vi "Stream Controller (FPGA).vi"() -> ()   [LabVIEW 2016]
doc: "Controls the generation and reception of data transferred from the Host to the FPGA.\nPort 0 receives data from the Port 0 TX Input DMA FIFO and transmits that data to Port 1.\nPort 1 receives data from the Port 1 TX Input DMA FIFO and transmits that data to Port 0."
uses:
  <instrlib>/_niInstr/Streaming/v1/Common/Stream State.ctl
  <vilib>/Platform/TimedLoop/XDataNode/timing_clust.ctl
  <vilib>/Platform/TimedLoop/XDataNode/nitl_modes.ctl
  <vilib>/Platform/TimedLoop/XDataNode/wakeup.ctl
  <instrlib>/_niInstr/CLIP Adapters/v1/FPGA/AXI4-Lite/FXP32 Address - FXP32 Data/Public/CLIP Resources.ctl
  <instrlib>/_niInstr/CLIP Adapters/v1/FPGA/AXI4-Lite/Address Space Collection/niInstr AXI4-Lite Address Space Collection v1 FPGA.lvclass
  C:/Program Files (x86)/National Instruments/LabVIEW 2016/instr.lib/_niInstr/Instruction Framework/v1/FPGA/Interfaces/Address Space Collection/Address Space Collection.lvclass
  <instrlib>/_niInstr/FIFO Register Bus/v1/FPGA/niInstr FIFO Register Bus v1 FPGA.lvclass
  C:/Program Files (x86)/National Instruments/LabVIEW 2016/instr.lib/_niInstr/Instruction Framework/v1/FPGA/Interfaces/Instruction Producer/Instruction Producer.lvclass
  <instrlib>/_niInstr/CLIP Adapters/v1/FPGA/AXI4-Stream/Reader FXP64x1/niInstr AXI4-Stream Reader FXP64x1 v1 FPGA.lvclass
  C:/Program Files (x86)/National Instruments/LabVIEW 2016/instr.lib/_niInstr/CLIP Adapters/v1/FPGA/AXI4-Stream/Reader/niInstr AXI4-Stream Reader v1 FPGA.lvclass
  <instrlib>/_niInstr/CLIP Adapters/v1/FPGA/AXI4-Stream/Writer FXP64x1/niInstr AXI4-Stream Writer FXP64x1 v1 FPGA.lvclass
  C:/Program Files (x86)/National Instruments/LabVIEW 2016/instr.lib/_niInstr/CLIP Adapters/v1/FPGA/AXI4-Stream/Writer/niInstr AXI4-Stream Writer v1 FPGA.lvclass
  <vilib>/rvi/Emulation/niFpgaSctlEmulationGetInTimedLoop.vi
  <vilib>/rvi/Emulation/niFpgaEmulationReportErrorSimple.vi
  <vilib>/rvi/Emulation/niFpgaGetClockAttributes.vi
  <vilib>/rvi/Emulation/niFpgaCriticalErrorInLSC.vi
  <instrlib>/_niInstr/Basic Elements/v1/FPGA/Private/Read U64 FIFO.vi
  <instrlib>/_niInstr/Basic Elements/v1/FPGA/Private/Write U64 FIFO.vi
  <vilib>/rvi/Emulation/niFpgaProcessEmulError.vi
  <vilib>/rvi/eio/common/nirviEmuTemplateMethod_errors.vi
  <vilib>/Platform/TimedLoop/XDataNode/XDataNode.xnode
  <vilib>/eio/EIONode/EIONode.xnode
  <vilib>/Platform/TimedLoop/XDataNode/XDNodeRunTimeDep.lvlib
  <instrlib>/_niInstr/CLIP Adapters/v1/FPGA/AXI4-Stream/Writer/niInstr AXI4-Stream Writer v1 FPGA.lvclass
  <instrlib>/_niInstr/CLIP Adapters/v1/FPGA/AXI4-Stream/Reader/niInstr AXI4-Stream Reader v1 FPGA.lvclass
  <instrlib>/_niInstr/Basic Elements/v1/FPGA/niInstr Basic Elements v1 FPGA.lvlib
  SubVIS/Aurora Stream (NI 6592R) (FPGA).lvlib
  <instrlib>/_niInstr/Streaming/v1/FPGA/niInstr Streaming v1 FPGA.lvlib
  <instrlib>/_niInstr/Streaming/v1/Common/niInstr Streaming v1 Common.lvlib
  <instrlib>/_niInstr/Instruction Framework/v1/FPGA/Top Level Bus/Register Configuration/Register Configuration.lvclass
  <instrlib>/_niInstr/CLIP Adapters/v1/FPGA/AXI4-Lite/FXP32 Address - FXP32 Data/niInstr AXI4-Lite - FXP32 Address - FXP32 Data v1 FPGA.lvclass
panel:
  out "Er.Port 3":u32
  out "Er.Port 2":u32
  out "Er.Port 1":u32
  out "Er.Port 0":u32
  in  "Simulated data":bool
  in  "Reset":bool
  out "Port 3 Link Reset":bool
  out "Port 1 Link Reset":bool
  in  "Port 3 PMA Init":bool
  in  "Port 1 PMA Init":bool
  out "fifo reg bus data 0":u64
  out "fifo reg bus status 0":u32
  in  "fifo reg bus ctrl 0":u32
  in  "Port 0 PMA Init":bool
  in  "Port 2 PMA Init":bool
  out "Port 0 Debug Info":T1
  out "Port 0 Link Reset":bool
  out "Port 2 Link Reset":bool
  out "sFrontEndConfig_Complete":bool
  out "Port 2 Debug Info":T1
  out "stream.state 5":T2
  out "stream.samples transferred 5":u64
  out "stream.metadata 5":u64
  in  "stream.num samples 5":u64
  in  "stream.request state 5":T2
  out "stream.state 4":T2
  out "stream.samples transferred 4":u64
  out "stream.metadata 4":u64
  in  "stream.num samples 4":u64
  in  "stream.request state 4":T2
  in  "stream.request state 0":T2
  in  "stream.num samples 0":u64
  out "stream.metadata 0":u64
  out "stream.samples transferred 0":u64
  out "stream.state 0":T2
  in  "stream.num samples 1":u64
  in  "stream.request state 1":T2
  out "stream.state 1":T2
  out "stream.samples transferred 1":u64
  out "stream.metadata 1":u64
  in  "stream.request state 6":T2
  in  "stream.num samples 6":u64
  out "stream.metadata 6":u64
  out "stream.samples transferred 6":u64
  out "stream.state 6":T2
  in  "stream.request state 7":T2
  in  "stream.num samples 7":u64
  out "stream.metadata 7":u64
  out "stream.samples transferred 7":u64
  out "stream.state 7":T2
  out "Port 3 Debug Info":T1
  in  "stream.request state 2":T2
  in  "stream.num samples 2":u64
  out "stream.metadata 2":u64
  out "stream.samples transferred 2":u64
  out "stream.state 2":T2
  in  "stream.request state 3":T2
  in  "stream.num samples 3":u64
  out "stream.metadata 3":u64
  out "stream.samples transferred 3":u64
  out "stream.state 3":T2
  out "Port 1 Debug Info":T1
  # "Port 0"
  # "Port 1"
  # "Port 2"
  # "Port 3"
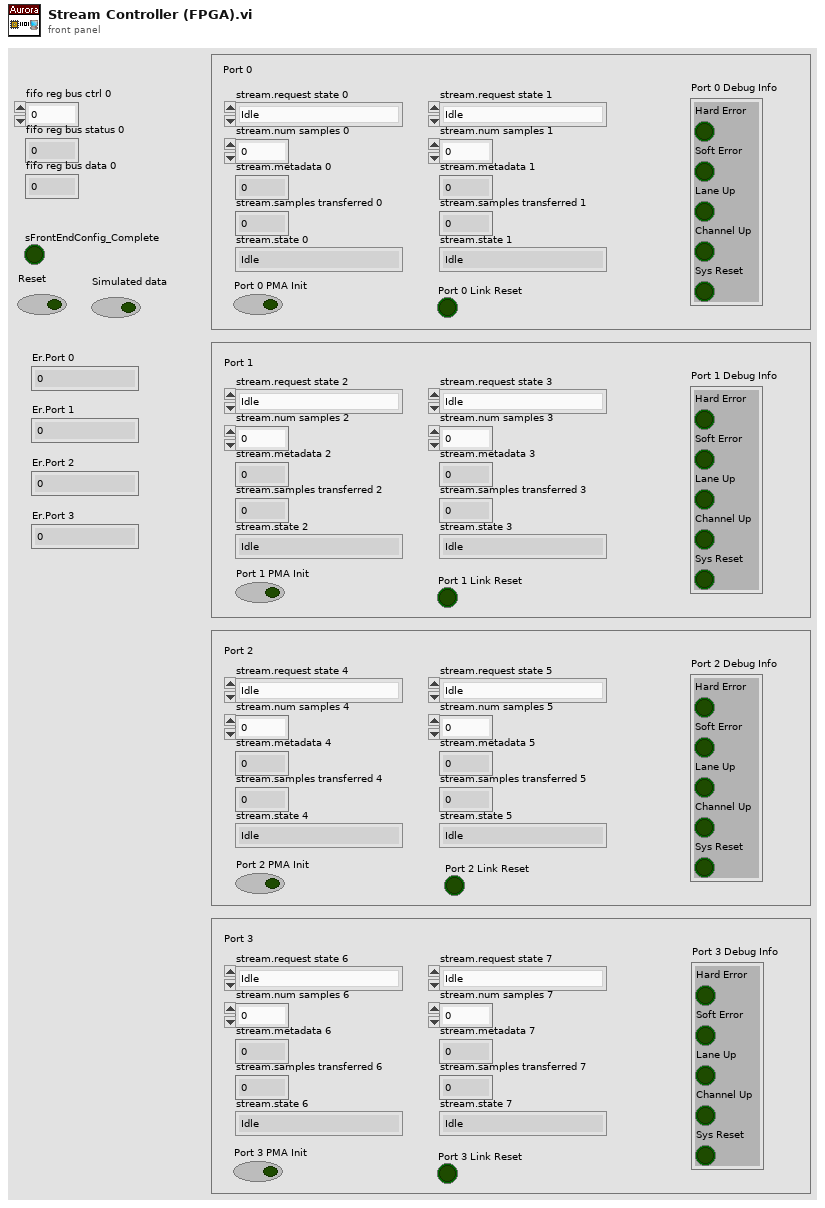
[diagram p1: front panel]
types:
  T1 = cluster{"Hard Error":bool, "Soft Error":bool, "Lane Up":bool, "Channel Up":bool, "Sys Reset":bool}
  T2 = typedef "niInstr Streaming v1 Common.lvlib/Stream State.ctl" = enum8{"Idle", "Finite Transfer", "Continuous", "Done", "Error", "Not Ready", "Cancel"}
  T3 = cluster{"Hard Error":refnum<k21>, "Soft Error":refnum<k21>, "Lane Up":refnum<k21>, "Channel Up":refnum<k21>, "Sys Reset":refnum<k21>}
  T4 = cluster{"m_axis_tvalid":refnum<k21>, "m_axis_tdata":refnum<k21>}
  T5 = cluster{"s_axis_tvalid":refnum<k21>, "s_axis_tdata":refnum<k21>, "s_axis_tready":refnum<k21>}
  T6 = typedef "niInstr AXI4-Lite - FXP32 Address - FXP32 Data v1 FPGA.lvclass/CLIP Resources.ctl" = cluster{"s_axi_araddr":refnum<k21>, "s_axi_arvalid":refnum<k21>, "s_axi_arready":refnum<k21>, "s_axi_rdata":refnum<k21>, "s_axi_rresp":refnum<k21>, "s_axi_rvalid":refnum<k21>, "s_axi_rready":refnum<k21>, "s_axi_awaddr":refnum<k21>, "s_axi_awvalid":refnum<k21>, "s_axi_awready":refnum<k21>, "s_axi_wdata":refnum<k21>, "s_axi_wstrb":refnum<k21>, "s_axi_wvalid":refnum<k21>, "s_axi_wready":refnum<k21>, "s_axi_bresp":refnum<k21>, "s_axi_bvalid":refnum<k21>, "s_axi_bready":refnum<k21>}
  T7 = typedef "XDNodeRunTimeDep.lvlib/timing_clust.ctl" = cluster{"Expected End [f-1]":u64, "Actual End [f-1]":u64, "Finished Late? [f-1]":bool, "Expected End [i-1]":u64, "Actual End [i-1]":u64, "Finished Late? [i-1]":bool, "Expected Start [i]":u64, "Actual Start [i]":u64, "Expected Start [f]":u64, "Actual Start [f]":u64, "Source Name":string, "Structure Name":string, "Period":i64, "Deadline":i64, "Offset":i64, "Start":i64, "Priority":i32, "Timeout":i32, "Mode":T8, "Wakeup Reason":T9, "Error":errorcluster, "Source Type":string, "Secondary Source Type":string, "Global End Time":u64, "Global Start Time":u64, "Frame Duration":u64, "Iteration Duration":u64, "Assigned CPU":i32, "I/O Scan Engine Mode":u32}
  T8 = typedef "XDNodeRunTimeDep.lvlib/nitl_modes.ctl" = enum32{"No Change", "Process missed periods, maintain original phase", "Discard missed periods, maintain original phase", "Process missed periods, ignore original phase", "Discard missed periods, ignore original phase"}
  T9 = typedef "XDNodeRunTimeDep.lvlib/wakeup.ctl" = enum32{"Normal", "Aborted", "Asynchronous wakeup", "Timing source error", "Timed loop error", "Timeout"}
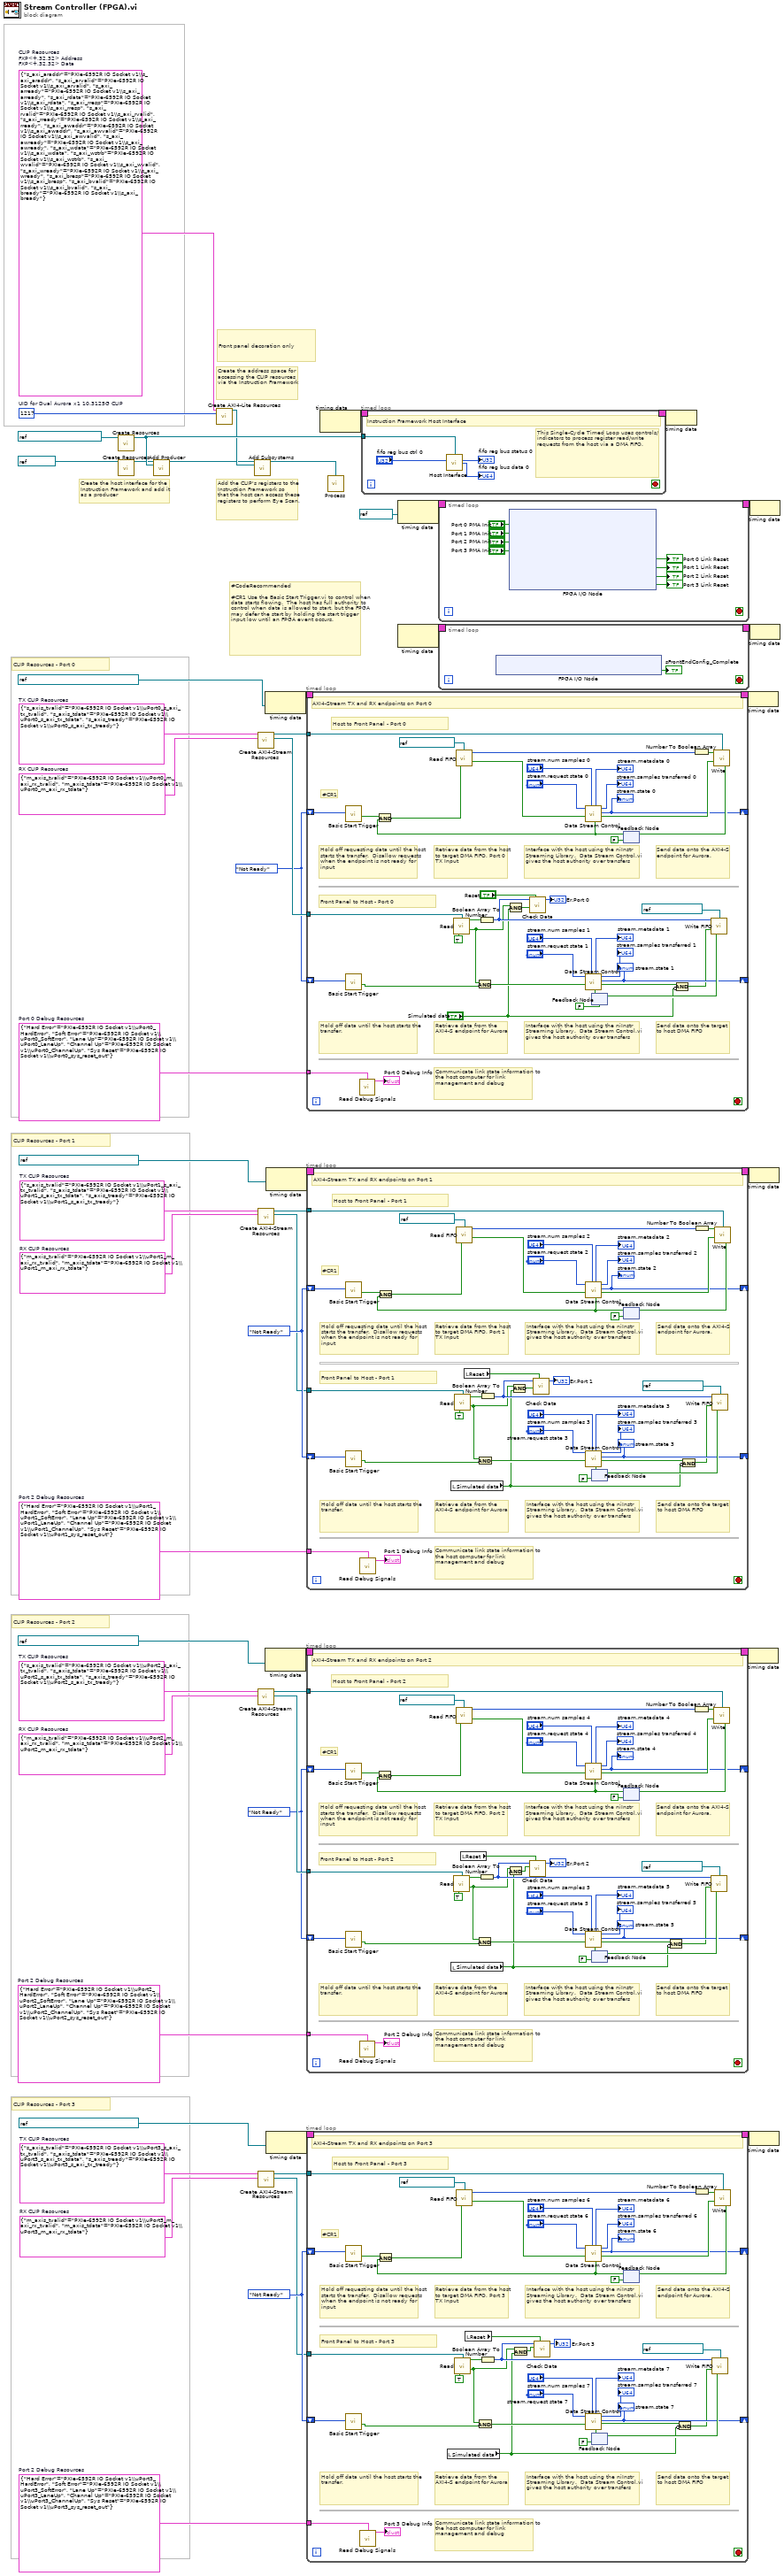
[diagram p0: block diagram]
diagram:
  w10 = T3 {"Hard Error"="PXIe-6592R IO Socket v1\\uPort3_HardError", "Soft Error"="PXIe-6592R IO Socket v1\\uPort3_SoftError", "Lane Up"="PXIe-6592R IO Socket v1\\uPort3_LaneUp", "Channel Up"="PXIe-6592R IO Socket v1\\uPort3_ChannelUp", "Sys Reset"="PXIe-6592R IO Socket v1\\uPort3_sys_reset_out"}  # Port 2 Debug Resources
  w9 = Stream_State."Not Ready" ("stream.state 0")
  w5 = T4 {"m_axis_tvalid"="PXIe-6592R IO Socket v1\\uPort3_m_axi_rx_tvalid", "m_axis_tdata"="PXIe-6592R IO Socket v1\\uPort3_m_axi_rx_tdata"}  # RX CLIP Resources
  w4 = T5 {"s_axis_tvalid"="PXIe-6592R IO Socket v1\\uPort3_s_axi_tx_tvalid", "s_axis_tdata"="PXIe-6592R IO Socket v1\\uPort3_s_axi_tx_tdata", "s_axis_tready"="PXIe-6592R IO Socket v1\\uPort3_s_axi_tx_tready"}  # TX CLIP Resources
  w19 = T3 {"Hard Error"="PXIe-6592R IO Socket v1\\uPort1_HardError", "Soft Error"="PXIe-6592R IO Socket v1\\uPort1_SoftError", "Lane Up"="PXIe-6592R IO Socket v1\\uPort1_LaneUp", "Channel Up"="PXIe-6592R IO Socket v1\\uPort1_ChannelUp", "Sys Reset"="PXIe-6592R IO Socket v1\\uPort1_sys_reset_out"}  # Port 2 Debug Resources
  w18 = Stream_State."Not Ready" ("stream.state 0")
  w14 = T4 {"m_axis_tvalid"="PXIe-6592R IO Socket v1\\uPort1_m_axi_rx_tvalid", "m_axis_tdata"="PXIe-6592R IO Socket v1\\uPort1_m_axi_rx_tdata"}  # RX CLIP Resources
  w13 = T5 {"s_axis_tvalid"="PXIe-6592R IO Socket v1\\uPort1_s_axi_tx_tvalid", "s_axis_tdata"="PXIe-6592R IO Socket v1\\uPort1_s_axi_tx_tdata", "s_axis_tready"="PXIe-6592R IO Socket v1\\uPort1_s_axi_tx_tready"}  # TX CLIP Resources
  w33 = u16 1217  # UID for Dual Aurora x1 10.3125G CLIP
  w34 = T6 {"s_axi_araddr"="PXIe-6592R IO Socket v1\\s_axi_araddr", "s_axi_arvalid"="PXIe-6592R IO Socket v1\\s_axi_arvalid", "s_axi_arready"="PXIe-6592R IO Socket v1\\s_axi_arready", "s_axi_rdata"="PXIe-6592R IO Socket v1\\s_axi_rdata", "s_axi_rresp"="PXIe-6592R IO Socket v1\\s_axi_rresp", "s_axi_rvalid"="PXIe-6592R IO Socket v1\\s_axi_rvalid", "s_axi_rready"="PXIe-6592R IO Socket v1\\s_axi_rready", "s_axi_awaddr"="PXIe-6592R IO Socket v1\\s_axi_awaddr", "s_axi_awvalid"="PXIe-6592R IO Socket v1\\s_axi_awvalid", "s_axi_awready"="PXIe-6592R IO Socket v1\\s_axi_awready", "s_axi_wdata"="PXIe-6592R IO Socket v1\\s_axi_wdata", "s_axi_wstrb"="PXIe-6592R IO Socket v1\\s_axi_wstrb", "s_axi_wvalid"="PXIe-6592R IO Socket v1\\s_axi_wvalid", "s_axi_wready"="PXIe-6592R IO Socket v1\\s_axi_wready", "s_axi_bresp"="PXIe-6592R IO Socket v1\\s_axi_bresp", "s_axi_bvalid"="PXIe-6592R IO Socket v1\\s_axi_bvalid", "s_axi_bready"="PXIe-6592R IO Socket v1\\s_axi_bready"}  # CLIP Resources FXP<+,32,32> Address FXP<+,32,32> Data
  w22 = T3 {"Hard Error"="PXIe-6592R IO Socket v1\\uPort2_HardError", "Soft Error"="PXIe-6592R IO Socket v1\\uPort2_SoftError", "Lane Up"="PXIe-6592R IO Socket v1\\uPort2_LaneUp", "Channel Up"="PXIe-6592R IO Socket v1\\uPort2_ChannelUp", "Sys Reset"="PXIe-6592R IO Socket v1\\uPort2_sys_reset_out"}  # Port 2 Debug Resources
  w40 = T3 {"Hard Error"="PXIe-6592R IO Socket v1\\uPort0_HardError", "Soft Error"="PXIe-6592R IO Socket v1\\uPort0_SoftError", "Lane Up"="PXIe-6592R IO Socket v1\\uPort0_LaneUp", "Channel Up"="PXIe-6592R IO Socket v1\\uPort0_ChannelUp", "Sys Reset"="PXIe-6592R IO Socket v1\\uPort0_sys_reset_out"}  # Port 0 Debug Resources
  w23 = Stream_State."Not Ready" ("stream.state 0")
  w41 = Stream_State."Not Ready" ("stream.state 0")
  w45 = T4 {"m_axis_tvalid"="PXIe-6592R IO Socket v1\\uPort2_m_axi_rx_tvalid", "m_axis_tdata"="PXIe-6592R IO Socket v1\\uPort2_m_axi_rx_tdata"}  # RX CLIP Resources
  w46 = T5 {"s_axis_tvalid"="PXIe-6592R IO Socket v1\\uPort2_s_axi_tx_tvalid", "s_axis_tdata"="PXIe-6592R IO Socket v1\\uPort2_s_axi_tx_tdata", "s_axis_tready"="PXIe-6592R IO Socket v1\\uPort2_s_axi_tx_tready"}  # TX CLIP Resources
  w47 = T4 {"m_axis_tvalid"="PXIe-6592R IO Socket v1\\uPort0_m_axi_rx_tvalid", "m_axis_tdata"="PXIe-6592R IO Socket v1\\uPort0_m_axi_rx_tdata"}  # RX CLIP Resources
  w48 = T5 {"s_axis_tvalid"="PXIe-6592R IO Socket v1\\uPort0_s_axi_tx_tvalid", "s_axis_tdata"="PXIe-6592R IO Socket v1\\uPort0_s_axi_tx_tdata", "s_axis_tready"="PXIe-6592R IO Socket v1\\uPort0_s_axi_tx_tready"}  # TX CLIP Resources
  # "CLIP Resources - Port 3"
  # "CLIP Resources - Port 1"
  # "CLIP Resources - Port 2"
  # "CLIP Resources - Port 0"
  # "#CodeRecommended\n\n#CR1 Use the Basic Start Trigger.vi to control when data starts flowing.  The host has full authority to control when data is allowed to start, but the FPGA may defer the start by holding the start trigger input low until an FPGA event occurs."
  # "Add the CLIP's registers to the Instruction Framework so\nthat the host can access these registers to perform Eye Scan."
  # "Create the host interface for the Instruction Framework and add it as a producer"
  # "Create the address space for accessing the CLIP resources via the Instruction Framework"
  # "Front panel decoration only"
  n1 = call <instrlib>:"Create Resources.vi"("instruction fifo"=refnum<k21> "reg.host instruction fifo 0" ("FIFO")) -> ("fifo register bus"=w35:refnum<class "niInstr FIFO Register Bus v1 FPGA.lvclass">)  [unwired: 14 in]
  n2 = call <instrlib>:"Create Resources.vi"("register clock"=refnum<k21> "100MHz" ("Source Name")) -> ("register configuration"=w31:refnum<class "Register Configuration.lvclass">)  [unwired: 14 in]
  n3 = call <instrlib>:"Add Producer.vi"("register configuration in"=w31, "instruction producer"=w35) -> ("register configuration out"=w30:refnum<class "Register Configuration.lvclass">)  [unwired: 13 in]
  n4 = call "Create AXI4-Lite Resources.vi"("CLIP Resources\nFXP<+,32,32> Address\nFXP<+,32,32> Data"=w34, "UID for Dual Aurora x1 10.3125G CLIP"=w33) -> ("niInstr AXI4-Lite Address Space Collection v1 FPGA out"=w32:refnum<class "niInstr AXI4-Lite Address Space Collection v1 FPGA.lvclass">)  [unwired: 13 in]
  n5 = call <instrlib>:"Add Subsystems.vi"("register configuration in"=w30, "subsystems"=w32) -> ("register configuration out"=w29:refnum<class "Register Configuration.lvclass">)  [unwired: 13 in]
  n6 = call "Create AXI4-Stream Resources.vi"("RX CLIP Resources"=w47, "TX CLIP Resources"=w48) -> ("RX niInstr AXI4-Stream Reader FXP64x1 v1 FPGA out"=w42:refnum<class "niInstr AXI4-Stream Reader FXP64x1 v1 FPGA.lvclass">, "TX niInstr AXI4-Stream Reader FXP64x1 v1 FPGA out"=w49:refnum<class "niInstr AXI4-Stream Writer FXP64x1 v1 FPGA.lvclass">)  [unwired: 8 in]
  n7 = call "Create AXI4-Stream Resources.vi"("RX CLIP Resources"=w45, "TX CLIP Resources"=w46) -> ("RX niInstr AXI4-Stream Reader FXP64x1 v1 FPGA out"=w24:refnum<class "niInstr AXI4-Stream Reader FXP64x1 v1 FPGA.lvclass">, "TX niInstr AXI4-Stream Reader FXP64x1 v1 FPGA out"=w25:refnum<class "niInstr AXI4-Stream Writer FXP64x1 v1 FPGA.lvclass">)  [unwired: 8 in]
  n8 = call "Create AXI4-Stream Resources.vi"("RX CLIP Resources"=w14, "TX CLIP Resources"=w13) -> ("RX niInstr AXI4-Stream Reader FXP64x1 v1 FPGA out"=w17:refnum<class "niInstr AXI4-Stream Reader FXP64x1 v1 FPGA.lvclass">, "TX niInstr AXI4-Stream Reader FXP64x1 v1 FPGA out"=w16:refnum<class "niInstr AXI4-Stream Writer FXP64x1 v1 FPGA.lvclass">)  [unwired: 8 in]
  n9 = call "Create AXI4-Stream Resources.vi"("RX CLIP Resources"=w5, "TX CLIP Resources"=w4) -> ("RX niInstr AXI4-Stream Reader FXP64x1 v1 FPGA out"=w8:refnum<class "niInstr AXI4-Stream Reader FXP64x1 v1 FPGA.lvclass">, "TX niInstr AXI4-Stream Reader FXP64x1 v1 FPGA out"=w7:refnum<class "niInstr AXI4-Stream Writer FXP64x1 v1 FPGA.lvclass">)  [unwired: 8 in]
  n10 = node-c288(refnum<k21> "PXIe-6592R IO Socket v1\\Port0_UserClk" ("Source Name")) -> (w52:T7)
  n11 = node-c288(refnum<k21> "PXIe-6592R IO Socket v1\\Port2_UserClk" ("Source Name")) -> (w28:T7)
  n12 = node-c288(refnum<k21> "PXIe-6592R IO Socket v1\\Port1_UserClk" ("Source Name")) -> (w21:T7)
  n13 = node-c288(refnum<k21> "PXIe-6592R IO Socket v1\\Port3_UserClk" ("Source Name")) -> (w12:T7)
  n14 = timed-loop {
    timing: w52 -> [_]
    timing-out: [_] -> w51
    tunnel: w49 -> [w93]
    tunnel: w42 -> [w92]
    shift-right: [w84] -> _
    shift-left: w41 -> [w79]
    shift-right: [w66] -> _
    shift-left: w41 -> [w72]
    tunnel: w40 -> [w64]
    stop <- _ stop-if-true
    # "#CR1"
    # "Communicate link state information to the host computer for link management and debug"
    # "Send data onto the target to host DMA FIFO"
    # "Interface with the host using the niInstr Streaming Library.  Data Stream Control.vi gives the host authority over transfers"
    # "Retrieve data from the AXI4-S endpoint for Aurora"
    # "Hold off data until the host starts the transfer."
    # "Send data onto the AXI4-S endpoint for Aurora."
    # "Interface with the host using the niInstr Streaming Library.  Data Stream Control.vi gives the host authority over transfers"
    # "Retrieve data from the host to target DMA FIFO, Port 0 TX Input"
    # "Hold off requesting data until the host starts the transfer.  Disallow requests when the endpoint is not ready for input"
    # "Front Panel to Host - Port 0"
    # "Host to Front Panel - Port 0"
    # "AXI4-Stream TX and RX endpoints on Port 0"
    n15 = call <instrlib>:"Basic Start Trigger.vi"("stream.state"=w79) -> ("data valid"=w78:bool)  [unwired: 10 in]
    n16 = call <instrlib>:"Basic Start Trigger.vi"("stream.state"=w72) -> ("data valid"=w71:bool)  [unwired: 10 in]
    n17 = call "Read Debug Signals.vi"("Debug CLIP Resources"=w64) -> ("Debug Info"=→"Port 0 Debug Info":T1)  [unwired: 14 in]
    n18 = call <instrlib>:"Read.vi"("niInstr AXI4-Stream Reader v1 FPGA in"=w92, "ready for output"=TRUE) -> ("tdata"=w88:bool[], "output valid"=w56:bool)  [unwired: 8 in, 4 out]
    n19 = And(x=w56, y=w71) -> (x .and. y?=w65:bool)
    n20 = Boolean Array To Number(Boolean array=w88) -> (number=w59:u64)
    n21 = Compound Arithmetic op=AND(w56, "Simulated data") -> (w55:bool)
    n22 = call "Check Data.vi"("reset"="Reset", "Input valid"=w55, "IQ Stream"=w59) -> ("errors"=→"Er.Port 0":u32)  [unwired: 8 in]
    n23 = feedback #1(FALSE ("ready for input")) -> (w73:bool)
    n24 = call <instrlib>:"Data Stream Control.vi"("ready for input?"=w73, "stream.num samples 0"="stream.num samples 1", "data valid"=w65, "stream.request state 0"="stream.request state 1") -> ("send data"=w58:bool, "stream.state 0"=w66:T2, "stream.samples transferred 0"=→"stream.samples transferred 1":u64, "stream.metadata 0"=→"stream.metadata 1":u64)  [unwired: 3 in, 1 out]
    "stream.state 1" <- w66
    n25 = feedback #2(FALSE ("ready for input")) -> (w77:bool)
    n26 = And(x=w78, y=w77) -> (x .and. y?=w76:bool)
    n27 = call-poly <instrlib>:"Read FIFO.vi"("fifo"=refnum<k21> "Port 0 TX Input", "ready for output"=w76) -> ("output data"=w86:u64, "output valid"=w75:bool)  [unwired: 12 in]
    n28 = call <instrlib>:"Data Stream Control.vi"("ready for input?"=w77, "stream.num samples 0"="stream.num samples 0", "data valid"=w75, "stream.request state 0"="stream.request state 0") -> ("send data"=w85:bool, "stream.state 0"=w84:T2, "stream.samples transferred 0"=→"stream.samples transferred 0":u64, "stream.metadata 0"=→"stream.metadata 0":u64)  [unwired: 3 in, 1 out]
    "stream.state 0" <- w84
    n29 = Compound Arithmetic op=AND(w58, invert "Simulated data") -> (w57:bool)
    n30 = Number To Boolean Array(number=w86) -> (Boolean array=w90:bool[])
    n31 = call-poly <instrlib>:"Write FIFO.vi"("input data"=w59, "fifo"=refnum<k21> "Port 0 RX Output", "input valid"=w57) -> ("ready for input"=w74:bool)  [unwired: 12 in]
    n32 = feedback-in #1(w74) -> ()
    n33 = call <instrlib>:"Write.vi"("tdata"=w90, "niInstr AXI4-Stream Writer v1 FPGA in"=w93, "input valid"=w85) -> ("ready for input"=w87:bool)  [unwired: 12 in]
    n34 = feedback-in #2(w87) -> ()
  }
  n35 = timed-loop {
    timing: w28 -> [_]
    timing-out: [_] -> w27
    tunnel: w25 -> [w137]
    tunnel: w24 -> [w136]
    shift-right: [w128] -> _
    shift-left: w23 -> [w123]
    shift-right: [w110] -> _
    shift-left: w23 -> [w116]
    tunnel: w22 -> [w108]
    stop <- _ stop-if-true
    # "#CR1"
    # "Communicate link state information to the host computer for link management and debug"
    # "Send data onto the target to host DMA FIFO"
    # "Interface with the host using the niInstr Streaming Library.  Data Stream Control.vi gives the host authority over transfers"
    # "Retrieve data from the AXI4-S endpoint for Aurora"
    # "Hold off data until the host starts the transfer."
    # "Send data onto the AXI4-S endpoint for Aurora."
    # "Interface with the host using the niInstr Streaming Library.  Data Stream Control.vi gives the host authority over transfers"
    # "Retrieve data from the host to target DMA FIFO, Port 2 TX Input"
    # "Hold off requesting data until the host starts the transfer.  Disallow requests when the endpoint is not ready for input"
    # "Front Panel to Host - Port 2"
    # "Host to Front Panel - Port 2"
    # "AXI4-Stream TX and RX endpoints on Port 2"
    n36 = call <instrlib>:"Basic Start Trigger.vi"("stream.state"=w123) -> ("data valid"=w122:bool)  [unwired: 10 in]
    n37 = call <instrlib>:"Basic Start Trigger.vi"("stream.state"=w116) -> ("data valid"=w115:bool)  [unwired: 10 in]
    n38 = call "Read Debug Signals.vi"("Debug CLIP Resources"=w108) -> ("Debug Info"=→"Port 2 Debug Info":T1)  [unwired: 14 in]
    n39 = local read "Simulated data"() -> (w98:bool)
    n40 = call <instrlib>:"Read.vi"("niInstr AXI4-Stream Reader v1 FPGA in"=w136, "ready for output"=TRUE) -> ("tdata"=w132:bool[], "output valid"=w101:bool)  [unwired: 8 in, 4 out]
    n41 = local read "Reset"() -> (w103:bool)
    n42 = And(x=w101, y=w115) -> (x .and. y?=w109:bool)
    n43 = Boolean Array To Number(Boolean array=w132) -> (number=w102:u64)
    n44 = Compound Arithmetic op=AND(w101, w98) -> (w100:bool)
    n45 = call "Check Data.vi"("reset"=w103, "Input valid"=w100, "IQ Stream"=w102) -> ("errors"=→"Er.Port 2":u32)  [unwired: 8 in]
    n46 = feedback #3(FALSE ("ready for input")) -> (w117:bool)
    n47 = call <instrlib>:"Data Stream Control.vi"("ready for input?"=w117, "stream.num samples 0"="stream.num samples 5", "data valid"=w109, "stream.request state 0"="stream.request state 5") -> ("send data"=w99:bool, "stream.state 0"=w110:T2, "stream.samples transferred 0"=→"stream.samples transferred 5":u64, "stream.metadata 0"=→"stream.metadata 5":u64)  [unwired: 3 in, 1 out]
    "stream.state 5" <- w110
    n48 = feedback #4(FALSE ("ready for input")) -> (w121:bool)
    n49 = And(x=w122, y=w121) -> (x .and. y?=w120:bool)
    n50 = call-poly <instrlib>:"Read FIFO.vi"("fifo"=refnum<k21> "Port 2 TX Input", "ready for output"=w120) -> ("output data"=w130:u64, "output valid"=w119:bool)  [unwired: 12 in]
    n51 = call <instrlib>:"Data Stream Control.vi"("ready for input?"=w121, "stream.num samples 0"="stream.num samples 4", "data valid"=w119, "stream.request state 0"="stream.request state 4") -> ("send data"=w129:bool, "stream.state 0"=w128:T2, "stream.samples transferred 0"=→"stream.samples transferred 4":u64, "stream.metadata 0"=→"stream.metadata 4":u64)  [unwired: 3 in, 1 out]
    "stream.state 4" <- w128
    n52 = Compound Arithmetic op=AND(w99, invert w98) -> (w97:bool)
    n53 = Number To Boolean Array(number=w130) -> (Boolean array=w134:bool[])
    n54 = call-poly <instrlib>:"Write FIFO.vi"("input data"=w102, "fifo"=refnum<k21> "Port 2 RX Output", "input valid"=w97) -> ("ready for input"=w118:bool)  [unwired: 12 in]
    n55 = feedback-in #3(w118) -> ()
    n56 = call <instrlib>:"Write.vi"("tdata"=w134, "niInstr AXI4-Stream Writer v1 FPGA in"=w137, "input valid"=w129) -> ("ready for input"=w131:bool)  [unwired: 12 in]
    n57 = feedback-in #4(w131) -> ()
  }
  n58 = timed-loop {
    timing: w21 -> [_]
    timing-out: [_] -> w20
    tunnel: w16 -> [w181]
    tunnel: w17 -> [w180]
    shift-right: [w172] -> _
    shift-left: w18 -> [w167]
    shift-right: [w154] -> _
    shift-left: w18 -> [w160]
    tunnel: w19 -> [w152]
    stop <- _ stop-if-true
    # "#CR1"
    # "Communicate link state information to the host computer for link management and debug"
    # "Send data onto the target to host DMA FIFO"
    # "Interface with the host using the niInstr Streaming Library.  Data Stream Control.vi gives the host authority over transfers"
    # "Retrieve data from the AXI4-S endpoint for Aurora"
    # "Hold off data until the host starts the transfer."
    # "Send data onto the AXI4-S endpoint for Aurora."
    # "Interface with the host using the niInstr Streaming Library.  Data Stream Control.vi gives the host authority over transfers"
    # "Retrieve data from the host to target DMA FIFO, Port 1 TX Input"
    # "Hold off requesting data until the host starts the transfer.  Disallow requests when the endpoint is not ready for input"
    # "Front Panel to Host - Port 1"
    # "Host to Front Panel - Port 1"
    # "AXI4-Stream TX and RX endpoints on Port 1"
    n59 = call <instrlib>:"Basic Start Trigger.vi"("stream.state"=w167) -> ("data valid"=w166:bool)  [unwired: 10 in]
    n60 = call <instrlib>:"Basic Start Trigger.vi"("stream.state"=w160) -> ("data valid"=w159:bool)  [unwired: 10 in]
    n61 = call "Read Debug Signals.vi"("Debug CLIP Resources"=w152) -> ("Debug Info"=→"Port 1 Debug Info":T1)  [unwired: 14 in]
    n62 = local read "Simulated data"() -> (w141:bool)
    n63 = call <instrlib>:"Read.vi"("niInstr AXI4-Stream Reader v1 FPGA in"=w180, "ready for output"=TRUE) -> ("tdata"=w176:bool[], "output valid"=w144:bool)  [unwired: 8 in, 4 out]
    n64 = local read "Reset"() -> (w146:bool)
    n65 = And(x=w144, y=w159) -> (x .and. y?=w153:bool)
    n66 = Boolean Array To Number(Boolean array=w176) -> (number=w145:u64)
    n67 = Compound Arithmetic op=AND(w144, w141) -> (w148:bool)
    n68 = call "Check Data.vi"("reset"=w146, "Input valid"=w148, "IQ Stream"=w145) -> ("errors"=→"Er.Port 1":u32)  [unwired: 8 in]
    n69 = feedback #5(FALSE ("ready for input")) -> (w161:bool)
    n70 = call <instrlib>:"Data Stream Control.vi"("ready for input?"=w161, "stream.num samples 0"="stream.num samples 3", "data valid"=w153, "stream.request state 0"="stream.request state 3") -> ("send data"=w143:bool, "stream.state 0"=w154:T2, "stream.samples transferred 0"=→"stream.samples transferred 3":u64, "stream.metadata 0"=→"stream.metadata 3":u64)  [unwired: 3 in, 1 out]
    "stream.state 3" <- w154
    n71 = feedback #6(FALSE ("ready for input")) -> (w165:bool)
    n72 = And(x=w166, y=w165) -> (x .and. y?=w164:bool)
    n73 = call-poly <instrlib>:"Read FIFO.vi"("fifo"=refnum<k21> "Port 1 TX Input", "ready for output"=w164) -> ("output data"=w174:u64, "output valid"=w163:bool)  [unwired: 12 in]
    n74 = call <instrlib>:"Data Stream Control.vi"("ready for input?"=w165, "stream.num samples 0"="stream.num samples 2", "data valid"=w163, "stream.request state 0"="stream.request state 2") -> ("send data"=w173:bool, "stream.state 0"=w172:T2, "stream.samples transferred 0"=→"stream.samples transferred 2":u64, "stream.metadata 0"=→"stream.metadata 2":u64)  [unwired: 3 in, 1 out]
    "stream.state 2" <- w172
    n75 = Compound Arithmetic op=AND(w143, invert w141) -> (w142:bool)
    n76 = Number To Boolean Array(number=w174) -> (Boolean array=w178:bool[])
    n77 = call-poly <instrlib>:"Write FIFO.vi"("input data"=w145, "fifo"=refnum<k21> "Port 1 RX Output", "input valid"=w142) -> ("ready for input"=w162:bool)  [unwired: 12 in]
    n78 = feedback-in #5(w162) -> ()
    n79 = call <instrlib>:"Write.vi"("tdata"=w178, "niInstr AXI4-Stream Writer v1 FPGA in"=w181, "input valid"=w173) -> ("ready for input"=w175:bool)  [unwired: 12 in]
    n80 = feedback-in #6(w175) -> ()
  }
  n81 = timed-loop {
    timing: w12 -> [_]
    timing-out: [_] -> w11
    tunnel: w7 -> [w225]
    tunnel: w8 -> [w224]
    shift-right: [w216] -> _
    shift-left: w9 -> [w211]
    shift-right: [w198] -> _
    shift-left: w9 -> [w204]
    tunnel: w10 -> [w196]
    stop <- _ stop-if-true
    # "#CR1"
    # "Communicate link state information to the host computer for link management and debug"
    # "Send data onto the target to host DMA FIFO"
    # "Interface with the host using the niInstr Streaming Library.  Data Stream Control.vi gives the host authority over transfers"
    # "Retrieve data from the AXI4-S endpoint for Aurora"
    # "Hold off data until the host starts the transfer."
    # "Send data onto the AXI4-S endpoint for Aurora."
    # "Interface with the host using the niInstr Streaming Library.  Data Stream Control.vi gives the host authority over transfers"
    # "Retrieve data from the host to target DMA FIFO, Port 3 TX Input"
    # "Hold off requesting data until the host starts the transfer.  Disallow requests when the endpoint is not ready for input"
    # "Front Panel to Host - Port 3"
    # "Host to Front Panel - Port 3"
    # "AXI4-Stream TX and RX endpoints on Port 3"
    n82 = call <instrlib>:"Basic Start Trigger.vi"("stream.state"=w211) -> ("data valid"=w210:bool)  [unwired: 10 in]
    n83 = call <instrlib>:"Basic Start Trigger.vi"("stream.state"=w204) -> ("data valid"=w203:bool)  [unwired: 10 in]
    n84 = call "Read Debug Signals.vi"("Debug CLIP Resources"=w196) -> ("Debug Info"=→"Port 3 Debug Info":T1)  [unwired: 14 in]
    n85 = local read "Simulated data"() -> (w186:bool)
    n86 = call <instrlib>:"Read.vi"("niInstr AXI4-Stream Reader v1 FPGA in"=w224, "ready for output"=TRUE) -> ("tdata"=w220:bool[], "output valid"=w189:bool)  [unwired: 8 in, 4 out]
    n87 = local read "Reset"() -> (w191:bool)
    n88 = And(x=w189, y=w203) -> (x .and. y?=w197:bool)
    n89 = Boolean Array To Number(Boolean array=w220) -> (number=w190:u64)
    n90 = Compound Arithmetic op=AND(w189, w186) -> (w188:bool)
    n91 = call "Check Data.vi"("reset"=w191, "Input valid"=w188, "IQ Stream"=w190) -> ("errors"=→"Er.Port 3":u32)  [unwired: 8 in]
    n92 = feedback #7(FALSE ("ready for input")) -> (w205:bool)
    n93 = call <instrlib>:"Data Stream Control.vi"("ready for input?"=w205, "stream.num samples 0"="stream.num samples 7", "data valid"=w197, "stream.request state 0"="stream.request state 7") -> ("send data"=w187:bool, "stream.state 0"=w198:T2, "stream.samples transferred 0"=→"stream.samples transferred 7":u64, "stream.metadata 0"=→"stream.metadata 7":u64)  [unwired: 3 in, 1 out]
    "stream.state 7" <- w198
    n94 = feedback #8(FALSE ("ready for input")) -> (w209:bool)
    n95 = And(x=w210, y=w209) -> (x .and. y?=w208:bool)
    n96 = call-poly <instrlib>:"Read FIFO.vi"("fifo"=refnum<k21> "Port 3 TX Input", "ready for output"=w208) -> ("output data"=w218:u64, "output valid"=w207:bool)  [unwired: 12 in]
    n97 = call <instrlib>:"Data Stream Control.vi"("ready for input?"=w209, "stream.num samples 0"="stream.num samples 6", "data valid"=w207, "stream.request state 0"="stream.request state 6") -> ("send data"=w217:bool, "stream.state 0"=w216:T2, "stream.samples transferred 0"=→"stream.samples transferred 6":u64, "stream.metadata 0"=→"stream.metadata 6":u64)  [unwired: 3 in, 1 out]
    "stream.state 6" <- w216
    n98 = Compound Arithmetic op=AND(w187, invert w186) -> (w185:bool)
    n99 = Number To Boolean Array(number=w218) -> (Boolean array=w222:bool[])
    n100 = call-poly <instrlib>:"Write FIFO.vi"("input data"=w190, "fifo"=refnum<k21> "Port 3 RX Output", "input valid"=w185) -> ("ready for input"=w206:bool)  [unwired: 12 in]
    n101 = feedback-in #7(w206) -> ()
    n102 = call <instrlib>:"Write.vi"("tdata"=w222, "niInstr AXI4-Stream Writer v1 FPGA in"=w225, "input valid"=w217) -> ("ready for input"=w219:bool)  [unwired: 12 in]
    n103 = feedback-in #8(w219) -> ()
  }
  n104 = node-c288() -> (w39:T7)  [unwired: 1 in]
  n105 = call <instrlib>:"Process.vi"("register configuration"=w29) -> ()  [unwired: 15 in]
  n106 = timed-loop {
    timing: w39 -> [_]
    timing-out: [_] -> w38
    tunnel: w35 -> [w229]
    stop <- _ stop-if-true
    # "This Single-Cycle Timed Loop uses controls/indicators to process register read/write requests from the host via a DMA FIFO."
    # "Instruction Framework Host Interface"
    n107 = call <instrlib>:"Host Interface.vi"("fifo register bus"=w229, "fifo reg bus ctrl 0"="fifo reg bus ctrl 0") -> ("fifo reg bus status 0"=→"fifo reg bus status 0":u32, "fifo reg bus data 0"=→"fifo reg bus data 0":u64)  [unwired: 12 in]
  }
  n108 = node-c288(refnum<k21> "50MHz" ("Source Name")) -> (w44:T7)
  n109 = node-c288() -> (w3:T7)  [unwired: 1 in]
  n110 = timed-loop {
    timing: w44 -> [_]
    timing-out: [_] -> w43
    stop <- _ stop-if-true
    n111 = xnode "FPGA I/O Node"("PXIe-6592R IO Socket v1\\cPort0_PMA_Init"="Port 0 PMA Init", "PXIe-6592R IO Socket v1\\cPort1_PMA_Init"="Port 1 PMA Init", "PXIe-6592R IO Socket v1\\cPort2_PMA_Init"="Port 2 PMA Init", "PXIe-6592R IO Socket v1\\cPort3_PMA_Init"="Port 3 PMA Init") -> ("PXIe-6592R IO Socket v1\\cPort0_link_reset_out"=→"Port 0 Link Reset":bool, "PXIe-6592R IO Socket v1\\cPort1_link_reset_out"=→"Port 1 Link Reset":bool, "PXIe-6592R IO Socket v1\\cPort2_link_reset_out"=→"Port 2 Link Reset":bool, "PXIe-6592R IO Socket v1\\cPort3_link_reset_out"=→"Port 3 Link Reset":bool)  [unwired: 8 in, 8 out]
  }
  n112 = timed-loop {
    timing: w3 -> [_]
    timing-out: [_] -> w2
    stop <- _ stop-if-true
    n113 = xnode "FPGA I/O Node"() -> ("PXIe-6592R IO Socket v1\\sFrontEndConfig_Complete"=→"sFrontEndConfig_Complete":bool)  [unwired: 1 in, 1 out]
  }
  n114 = node-c288(w38) -> ()
  n115 = node-c288(w51) -> ()
  n116 = node-c288(w27) -> ()
  n117 = node-c288(w20) -> ()
  n118 = node-c288(w11) -> ()
  n119 = node-c288(w43) -> ()
  n120 = node-c288(w2) -> ()
